vi "Get All Messages.vi"(8 "error in":errorcluster, 11 "port in":T1 format="%.0x") -> (0 "error out":errorcluster, 2 "messages":T1[](array[typedef]) format="%.0x", 3 "port out":T1 format="%.0x")   [LabVIEW 2020, in "AIM MIL-STD-1553 Scripting.lvlib"]
doc: "Returns references to all <b>messages</b> within the <b>port in</b>."
uses:
  AIM MIL-STD-1553 Scripting.lvlib
  <vilib>/NI VeriStand/Custom Device API/Custom Device Item Ref.ctl
  Constants.vi
  <vilib>/NI VeriStand/Custom Device Tools/Custom Device Utility Library/NI VeriStand - Search for All Items by GUID.vi
  <vilib>/NI VeriStand/Custom Device Tools/Custom Device Utility Library/Custom Device Utility Library.lvlib
  <vilib>/NI VeriStand/Custom Device API/Custom Device API.lvlib
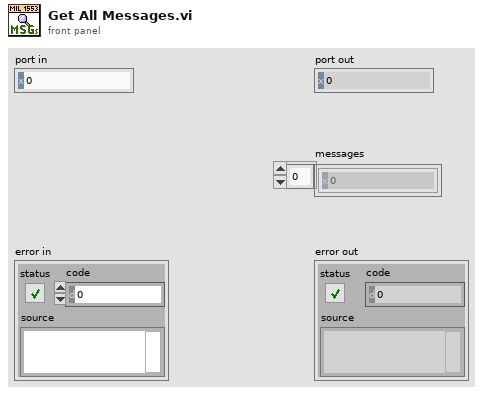
[diagram p1: front panel]
types:
  T1 = typedef "Custom Device API.lvlib/Custom Device Item Ref.ctl" = u64
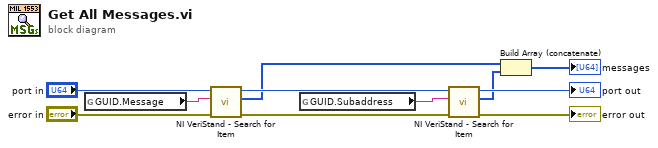
[diagram p0: block diagram]
diagram:
  n1 = global read "Constants.vi" "GUID.Message"() -> (w11:string)
  n2 = call-poly <vilib>:"NI VeriStand - Search for Item.vi"("error in"="error in", "Item GUID"=w11, "Section Ref in"="port in") -> ("error out"=w8:errorcluster, "Item Refs"=w3:T1[], "Section Ref out"=w7:T1)  [unwired: 5 in, 1 out]
  n3 = global read "Constants.vi" "GUID.Subaddress"() -> (w1:string)
  n4 = call-poly <vilib>:"NI VeriStand - Search for Item.vi"("error in"=w8, "Item GUID"=w1, "Section Ref in"=w7) -> ("error out"=→"error out":errorcluster, "Item Refs"=w4:T1[], "Section Ref out"=→"port out":T1)  [unwired: 5 in, 1 out]
  n5 = Build Array (concatenate)(w3, w4) -> (→"messages":T1[])
